vi "PKG_IMC_Setlimit.vi"(5 "axis":i32, 6 "nlimPolar":i32, 7 "nlimEna":i32, 9 "plimPolar":i32, 10 "plimEna":i32, 11 "handle":u32) -> (2 "function return":i32, 3 "handle out":u32)   [LabVIEW 2018, in "IMC_Pkg4xxx.lvlib"]
doc: "PKG_IMC_Setlimit (IMC_HANDLE handle, int plimEna, int plimPolar, int nlimEna, int nlimPolar, int axis);"
uses:
  IMC_Pkg4xxx.lvlib
  IMC_Pkg4xxx.dll
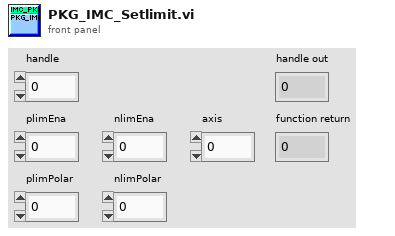
[diagram p1: front panel]
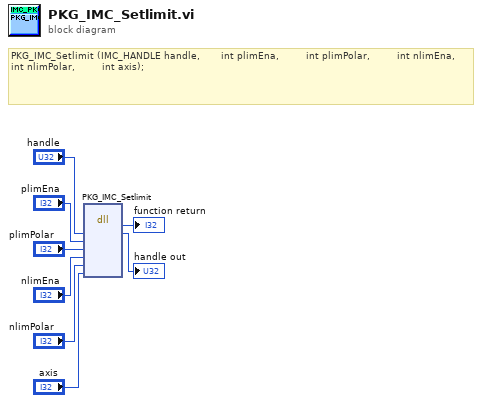
[diagram p0: block diagram]
diagram:
  # "PKG_IMC_Setlimit (IMC_HANDLE handle, \t\t\t\t\t\tint plimEna, \t\t\t\t\t\t\t\tint plimPolar, \t\t\t\t\t\t\t\tint nlimEna, \t\t\t\t\t\t\t\tint nlimPolar, \t\t\t\t\t\t\t\tint axis);"
  n1 = dll-call lib="PTH2\\abs D做的项目航天测量驱动电机IMCAppincLabview32\nIMC_Pkg4xxx.*" fn="PKG_IMC_Setlimit"("handle"="handle", "plimEna"="plimEna", "plimPolar"="plimPolar", "nlimEna"="nlimEna", "nlimPolar"="nlimPolar", "axis"="axis") -> (→"function return":i32, "handle"=→"handle out":u32)  [unwired: 8 in, 2 out]
